vi "Translate.vi"(10 "Message In":refnum<class "MSG.lvclass">, 11 "Translator in":refnum<class "Translator.lvclass">) -> (2 "Translated Message":refnum<class "MSG.lvclass">, 3 "Translator out":refnum<class "Translator.lvclass">)   [LabVIEW 2011, in "Messenging.lvlib" / "Translator.lvclass"]
uses:
  Translator.lvclass
  TextVarientMessage/MSG.lvclass
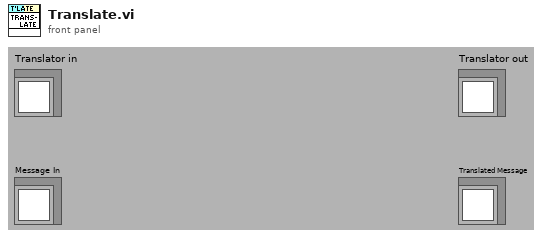
[diagram p1: front panel]
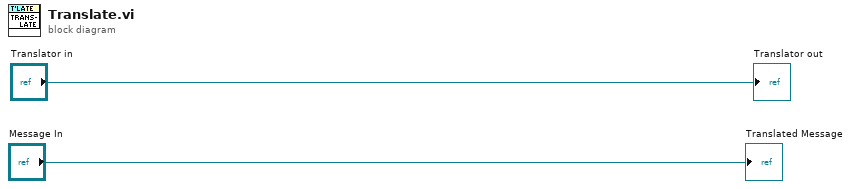
[diagram p0: block diagram]
diagram:
  "Translator out" <- "Translator in"
  "Translated Message" <- "Message In"
